vi "1.2signal_bruité_level02.vi"() -> ()   [LabVIEW 2018]
uses:
  <vilib>/measure/NI_MABase.lvlib
  <vilib>/Analysis/NI_AALBase.lvlib
panel:
  in  "Boolean":bool
  in  "nbr de signaux":dbl=3.0
  in  "stop":bool
  out "Waveform Graph":waveform(dbl)(graph)
  in  "Amplitude":dbl=1.0
  in  "Paramétre de siganl 2":T1={"Fréquence Echantioll"=1000.0, "nombre des echantionnage"=1000.0}
  in  "Paramétre de siganl":T2={"Amplitude"=1.0, "frequence"=2.0, "signal type"=enum."Sine Wave"}
  # "Bruit"
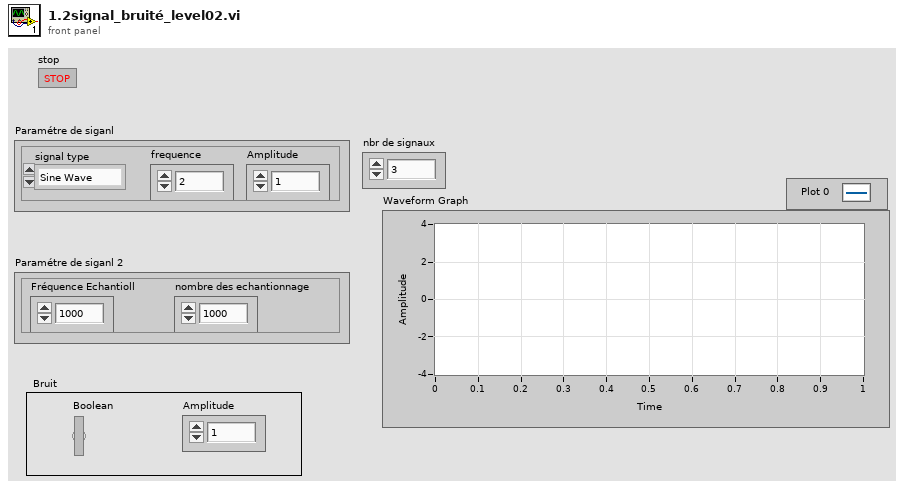
[diagram p1: front panel]
types:
  T1 = cluster{"Fréquence Echantioll":dbl, "nombre des echantionnage":dbl}
  T2 = cluster{"Amplitude":dbl, "frequence":dbl, "signal type":enum16{"Sine Wave", "Triangle Wave", "Square Wave", "Sawtooth Wave"}}
  T3 = enum16{"Sine Wave", "Triangle Wave", "Square Wave", "Sawtooth Wave"}
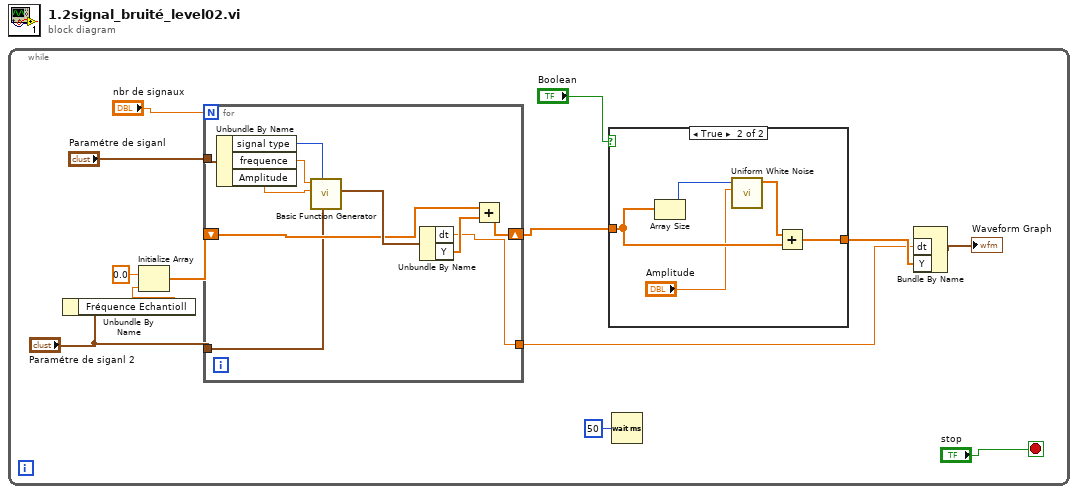
[diagram p0: block diagram]
diagram:
  n1 = while {
    stop <- "stop" stop-if-true
    n2 = Unbundle By Name("Paramétre de siganl 2") -> ("Fréquence Echantioll"=w11:dbl)
    n3 = Initialize Array(0.0 ("element"), w11) -> (w13:dbl[])
    n4 = for {
      N: "nbr de signaux" -> [_]
      shift-right: [w27] -> w9
      shift-left: w13 -> [w26]
      tunnel: "Paramétre de siganl 2" -> [w25]
      tunnel: [w24] -> w7
      tunnel: "Paramétre de siganl" -> [w20]
      n5 = Unbundle By Name(w20) -> ("signal type"=w23:T3, "frequence"=w22:dbl, "Amplitude"=w21:dbl)
      n6 = call <vilib>:"Basic Function Generator.vi"("sampling info"=w25, "signal type"=w23, "amplitude"=w21, "frequency"=w22) -> ("signal out"=w29:waveform(dbl))  [unwired: 5 in, 2 out]
      n7 = Unbundle By Name(w29) -> ("dt"=w24:dbl, "Y"=w28:dbl[])
      n8 = Add(x=w26, y=w28) -> (x+y=w27:dbl[])
    }
    n9 = case shown="True" "Boolean" {
      tunnel: w9 -> [w14 w17]
      tunnel: [w14 w15] -> w8
      frame False {
      }
      frame True {
        n10 = Array Size(array=w17) -> (size(s)=w19:i32)
        n11 = call <vilib>:"Uniform White Noise.vi"("amplitude"="Amplitude", "samples"=w19) -> ("uniform white noise"=w18:dbl[])  [unwired: 8 in, 1 out]
        n12 = Add(x=w18, y=w17) -> (x+y=w15:dbl[])
      }
    }
    n13 = Wait (ms)(milliseconds to wait=u32 50) -> ()  [unwired: 1 out]
    n14 = Bundle By Name("dt"=w7, "Y"=w8) -> (→"Waveform Graph":waveform(dbl))  [unwired: 1 in]
  }
